vi "Start Acquisition.vi"(8 "error in (no error)":errorcluster, 10 "Camera Name":string, 11 "IMAQdx Actor in":refnum<class "IMAQdx Actor.lvclass">) -> (0 "error out":errorcluster {"code" format="%.0x"}, 3 "IMAQdx Actor out":refnum<class "IMAQdx Actor.lvclass">)   [LabVIEW 2020, in "IMAQdx Actor.lvlib" / "IMAQdx Actor.lvclass"]
uses:
  IMAQdx Actor.lvclass
  C:/Users/AlexK/work/LabVIEW Programme/POLARIS CAM Log Abw und E/Submodules/HIJ Vision/Camera Actors/Camera Actor/Camera Actor/Camera Actor.lvclass
  Camera Actor/Camera Actor/Camera Actor.lvclass/Camera Actor.ctl
  <vilib>/vision/driver/IMAQdx.llb/IMAQdx Camera Control Mode.ctl
  <vilib>/vision/driver/IMAQdx.llb/IMAQdx Acquisition Mode.ctl
  Camera Actor/Camera Actor/Operation Mode.ctl
  IMAQdx Actor.lvclass/IMAQdx Actor.ctl
  Camera Actor/Camera Actor/Read Image ref.vi
  Camera Actor/Camera Actor/Write Camera Name.vi
  Camera Actor/Camera Actor/Write Image.vi
  Camera Actor/Camera Actor/Read Camera State.vi
  Camera Actor/Camera Actor/Camera Actor.lvclass
  <vilib>/vision/driver/NI_Vision_Acquisition_Software.lvlib
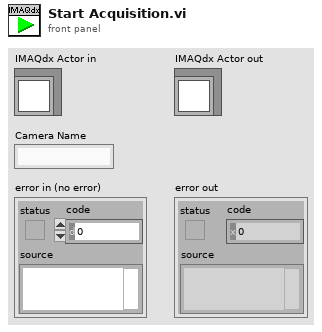
[diagram p1: front panel]
types:
  T1 = typedef "NI_Vision_Acquisition_Software.lvlib/IMAQdx Acquisition Mode.ctl" = enum32{"One Shot", "Continuous"}
  T2 = typedef "NI_Vision_Acquisition_Software.lvlib/IMAQdx Camera Control Mode.ctl" = enum32{"Controller", "Listener"}
  T3 = typedef "Camera Actor.lvlib/Camera Actor.lvclass/Operation Mode.ctl" = enum16{"Run", "Stop", "Exit", "Error", "Restart"}
  T4 = typedef "Image Type" = u32
  T5 = typedef "IMAQ Image.ctl" = refnum<image>
  T6 = typedef "IMAQdx.ctl" = refnum<k21>
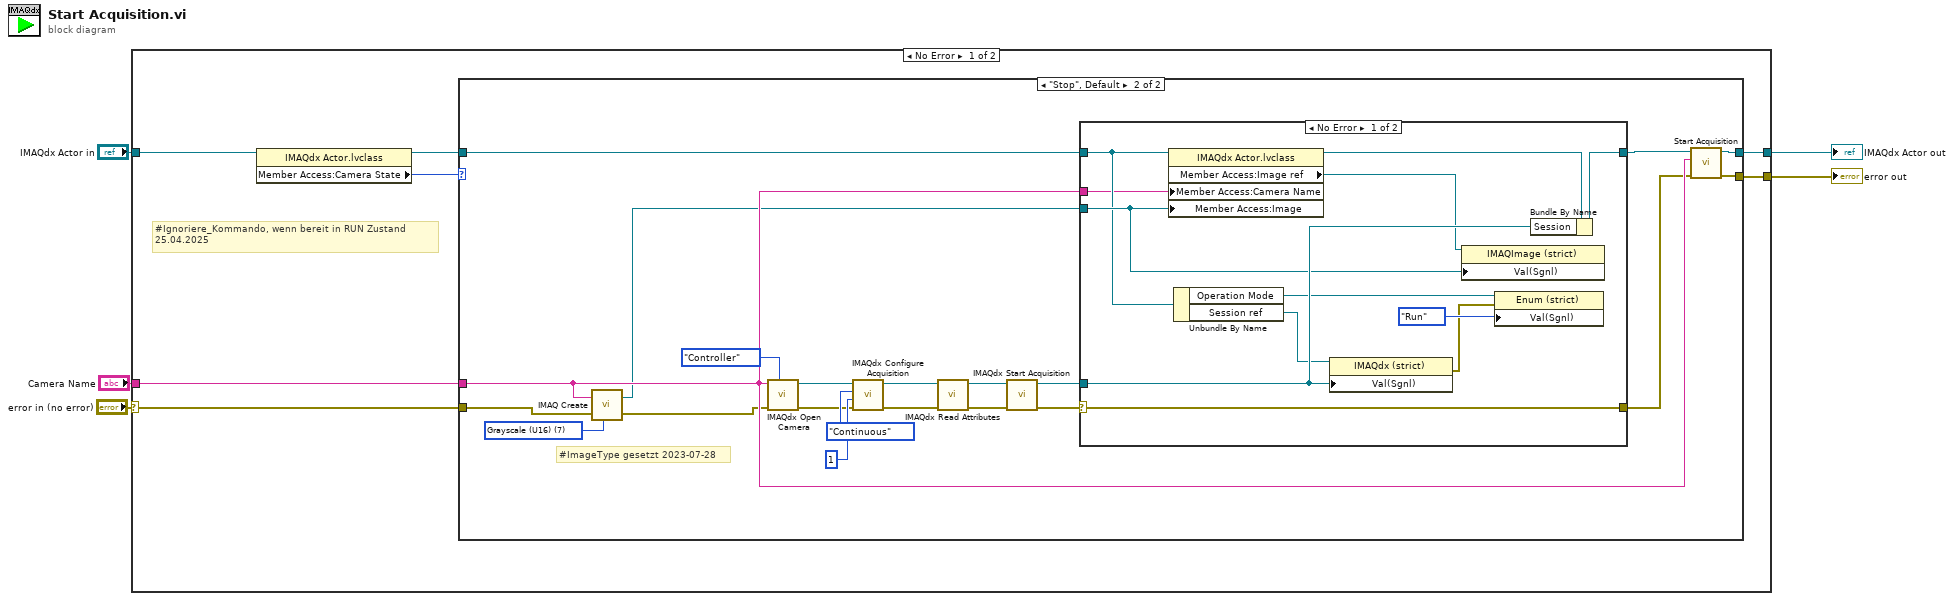
[diagram p0: block diagram]
diagram:
  n1 = case shown="No Error" "error in (no error)" {
    selector: "error in (no error)" -> [w12 w50]
    tunnel: "IMAQdx Actor in" -> [w11 w51]
    tunnel: "Camera Name" -> [w10 _]
    tunnel: [w9 w50] -> w2
    tunnel: [w8 w51] -> w1
    frame No Error {
      # "#Ignoriere_Kommando, wenn bereit in RUN Zustand\n25.04.2025"
      n2 = property class="IMAQdx Actor.lvclass"(reference=w11) -> (reference out=w7:refnum<class "IMAQdx Actor.lvclass">, "Member Access:Camera State"=w6:T3)  [unwired: 1 in, 1 out]
      n3 = case shown="\"Stop\", Default" w6 {
        tunnel: w12 -> [w13 w26]
        tunnel: w10 -> [_ w35]
        tunnel: [w13 w17] -> w9
        tunnel: [w14 w16] -> w8
        tunnel: w7 -> [w14 w15]
        frame "Run" {
        }
        frame "Stop", Default {
          w20 = T4 7 items=["Grayscale (U8)", "Grayscale (I16)", "Grayscale (SGL)", "Complex (CSG)", "RGB (U32)", "HSL (U32)", "RGB (U64)", "Grayscale (U16)"] ("Image Type")
          # "#ImageType gesetzt 2023-07-28"
          n4 = call "IMAQ Create"("Image Name"=w35, "Image Type"=w20, "error in (no error)"=w26) -> ("New Image"=w23:T5, "error out"=w28:errorcluster)  [unwired: 1 in, 1 out]
          n5 = call <vilib>:"IMAQdx Open Camera.vi"("Camera Control Mode"=IMAQdx_Camera_Control_Mode."Controller", "error in"=w28, "Session In"=w35) -> ("error out"=w29:errorcluster, "Session Out"=w27:T6)  [unwired: 7 out]
          n6 = call <vilib>:"IMAQdx Configure Acquisition.vi"("error in"=w29, "Number of Buffers"=u32 1, "Continuous?"=IMAQdx_Acquisition_Mode."Continuous", "Session In"=w27) -> ("error out"=w30:errorcluster, "Session Out"=w31:T6)  [unwired: 6 out]
          n7 = call <vilib>:"IMAQdx Read Attributes.vi"("error in"=w30, "Session In"=w31) -> ("error out"=w24:errorcluster, "Session Out"=w25:T6)  [unwired: 8 in]
          n8 = call <vilib>:"IMAQdx Start Acquisition.vi"("error in"=w24, "Session In"=w25) -> ("error out"=w22:errorcluster, "Session Out"=w21:T6)  [unwired: 8 out]
          n9 = case shown="No Error" w22 {
            selector: w22 -> [w42 w49]
            tunnel: w21 -> [w47 _]
            tunnel: w23 -> [w39 _]
            tunnel: w15 -> [w38 w48]
            tunnel: [w43 w48] -> w18
            tunnel: w35 -> [w36 _]
            tunnel: [w42 w49] -> w19
            frame No Error {
              n10 = property class="IMAQdx Actor.lvclass"(reference=w38, "Member Access:Camera Name"=w36, "Member Access:Image"=w39) -> (reference out=w41:refnum<class "IMAQdx Actor.lvclass">, "Member Access:Image ref"=w40:refnum<vi>)  [unwired: 1 in, 1 out]
              n11 = Unbundle By Name(w38) -> ("Operation Mode"=w45:refnum<vi>, "Session ref"=w46:refnum<vi>)
              n12 = property class="IMAQdx (strict)"(reference=w46, "Val(Sgnl)"=w47) -> (error out=w37:errorcluster)  [unwired: 1 in, 1 out]
              n13 = property class="IMAQImage (strict)"(reference=w40, "Val(Sgnl)"=w39) -> ()  [unwired: 1 in, 2 out]
              n14 = property class="Enum (strict)"(reference=w45, error in=w37, "Val(Sgnl)"=Operation_Mode."Run" ("Value (Signaling)")) -> ()  [unwired: 2 out]
              n15 = Bundle By Name(cluster=w41, "Session"=w47) -> (w43:refnum<class "IMAQdx Actor.lvclass">)
            }
            frame Error {
            }
          }
          n16 = call-parent "Start Acquisition.vi"("error in (no error)"=w19, "Camera Name"=w35, "Camera in"=w18) -> ("error out"=w17:errorcluster, "Camera out"=w16:refnum<class "IMAQdx Actor.lvclass">)  [unwired: 7 in]
        }
      }
    }
    frame Error {
    }
  }
  "error out" <- w2
  "IMAQdx Actor out" <- w1
